vi "Menu_Check.vi"(7 "Ctrl":string, 8 "error in (no error)":errorcluster, 10 "DB Ref":T1, 11 "String":string) -> (0 "error out":errorcluster)   [LabVIEW 2017, in "tagdb-RefMgr Operations.lvlib"]
uses:
  tagdb-RefMgr Operations.lvlib
  <userlib>/_NEVSTOP/TagDB/Typedef/TagDB.ctl
  00d0da00-135c-4b50-b029-f1f1f0d03544.vi
  4c542a80-f847-4821-836c-1c9f0a826a9d.vi
  00d0da00-135c-4b50-b029-f1f1f0d03544.vi/1b47866c-8e2d-43a7-815f-8cf18635e5a1.vi
  4c542a80-f847-4821-836c-1c9f0a826a9d.vi/1b47866c-8e2d-43a7-815f-8cf18635e5a1.vi
  <userlib>/_NEVSTOP/TagDB/_Support/Change Detector/TagDB dbChanged.vi
  <userlib>/_NEVSTOP/TagDB/_Support/Error/_Clear Errors.vi
  00d0da00-135c-4b50-b029-f1f1f0d03544.vi/1b47866c-8e2d-43a7-815f-8cf18635e5a1.vi/29b2ea6d-6d7f-4e4a-ad31-a5cb760462c7.vi
  <userlib>/_NEVSTOP/TagDB/API/TagDB-Status.vi
  4c542a80-f847-4821-836c-1c9f0a826a9d.vi/1b47866c-8e2d-43a7-815f-8cf18635e5a1.vi/29b2ea6d-6d7f-4e4a-ad31-a5cb760462c7.vi
  <userlib>/_NEVSTOP/TagDB/_Support/Change Detector/TagDB ChangeFlag.vi
  <userlib>/_NEVSTOP/TagDB/_Support/DataAccess/_NameCacher.vi
  <userlib>/_NEVSTOP/TagDB/_Support/Error/_[error50002]Invalid DataType.vi
  <userlib>/_NEVSTOP/TagDB/_Support/Error/_[error50000]Invalid DB REF.vi
  <userlib>/_NEVSTOP/TagDB/_Support/DataAccess/TagDB Ref to DVR.vi
  <userlib>/_NEVSTOP/TagDB/_Support/URL/TRIM-BOTH-SPACE.vi
  <userlib>/_NEVSTOP/TagDB/_Support/Error/_Build Error Cluster.vi
  <userlib>/_NEVSTOP/TagDB/TagDB.lvlib
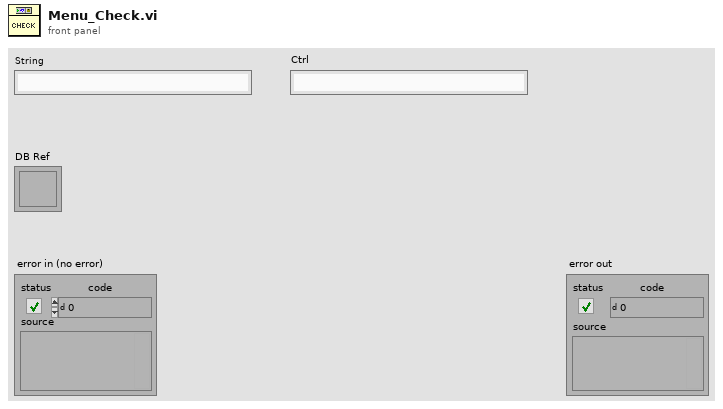
[diagram p1: front panel]
types:
  T1 = typedef "TagDB.lvlib/TagDB.ctl" = refnum<k1>
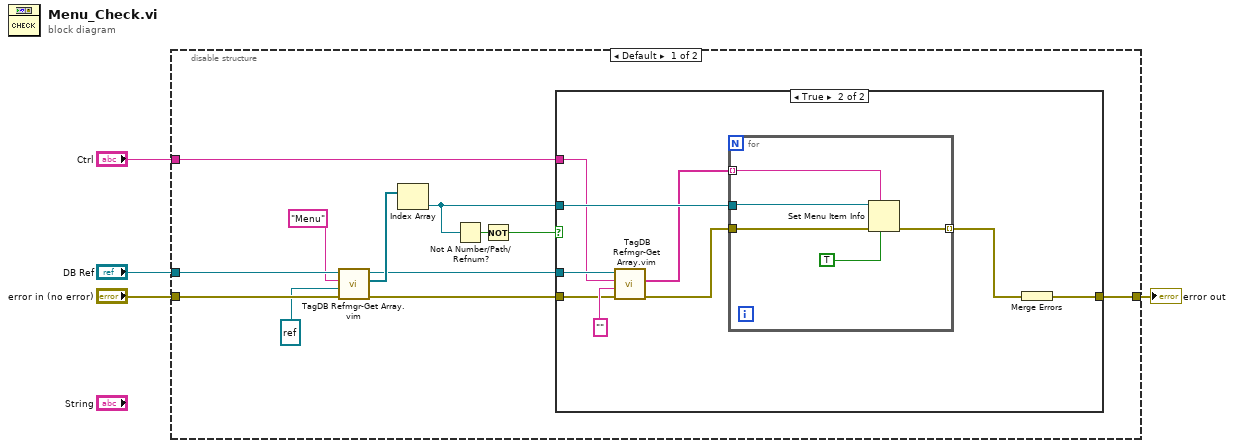
[diagram p0: block diagram]
diagram:
  n1 = disable-structure shown="Default" {
    disable-tunnel: "error in (no error)" -> [w16 w32]
    disable-tunnel: "DB Ref" -> [w15 _]
    disable-tunnel: "Ctrl" -> [w10 _]
    disable-tunnel: [w9 w32] -> w1
    frame condition #0 (active) {
      n2 = call "TagDB Refmgr-Get Array.vim"("error in (no error)"=w16, "Type"=refnum<k9> refnum ("menu reference"), "RegExp"="Menu", "DB Ref"=w15) -> ("error out"=w8:errorcluster, "References"=w12:refnum<k9>[], "DB Ref(dup)"=w11:T1)  [unwired: 4 in, 1 out]
      n3 = Index Array(array=w12) -> (element=w5:refnum<k9>)  [unwired: 1 in]
      n4 = Not A Number/Path/Refnum?(number/path/refnum=w5) -> (NaN/Path/Refnum?=w7:bool)
      n5 = Not(x=w7) -> (.not. x?=w6:bool)
      n6 = case shown="True" w6 {
        tunnel: w11 -> [_ w26]
        tunnel: w5 -> [_ w25]
        tunnel: w10 -> [_ w23]
        tunnel: [w17 w20] -> w9
        tunnel: w8 -> [w17 w19]
        frame False {
        }
        frame True {
          n7 = call "TagDB Refmgr-Get Array.vim"("error in (no error)"=w19, "Type"="" ("RegExp"), "RegExp"=w23, "DB Ref"=w26) -> ("error out"=w18:errorcluster, "References"=w22:string[])  [unwired: 4 in, 2 out]
          n8 = for {
            tunnel: w25 -> [w31]
            tunnel: w22 -> [w29] mode=indexing
            tunnel: w18 -> [w28]
            tunnel: [w27] -> w21 mode=indexing
            n9 = Set Menu Item Info(6:TRUE ("checked"), 7:w29, 8:w28, 11:w31) -> (0:w27:errorcluster)  [unwired: 3 in, 1 out]
          }
          n10 = Merge Errors(w21) -> (w20:errorcluster)
        }
      }
    }
    frame condition #1 {
    }
  }
  "error out" <- w1
